vi "Operate.vi"(8 "error in (no error)":errorcluster, 11 "Multiply in":refnum<class "Multiply.lvclass">) -> (0 "error out":errorcluster, 3 "Multiply out":refnum<class "Multiply.lvclass">)   [LabVIEW 2020, in "Multiply.lvclass"]
doc: "This method is used as a child which is used to perform multiplication operation"
uses:
  Multiply.lvclass
  D:/labview/Assignment 24/Math Operations/Math Operations.lvclass
  Multiply.lvclass/Multiply.ctl
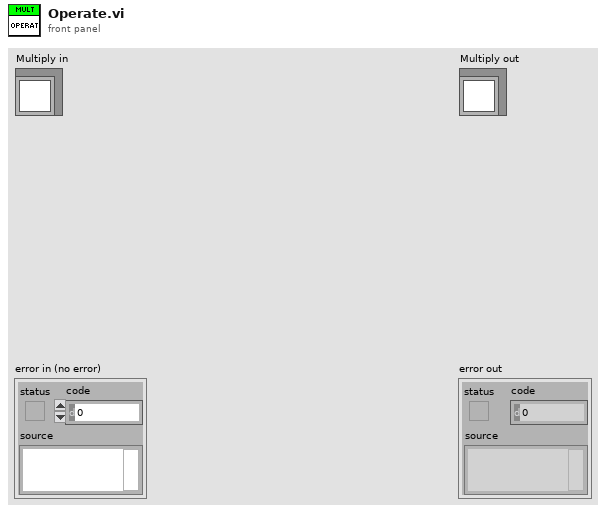
[diagram p1: front panel]
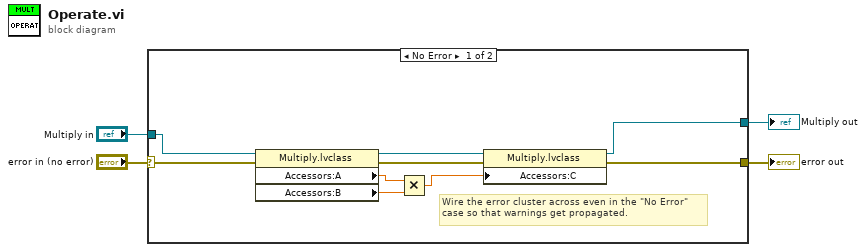
[diagram p0: block diagram]
diagram:
  n1 = case shown="No Error" "error in (no error)" {
    selector: "error in (no error)" -> [w13 w15]
    tunnel: [w6 w15] -> w3
    tunnel: [w5 w14] -> w1
    tunnel: "Multiply in" -> [w11 w14]
    frame No Error {
      # "Wire the error cluster across even in the \"No Error\"\ncase so that warnings get propagated."
      n2 = property class="Multiply.lvclass"(reference=w11, error in=w13) -> (reference out=w10:refnum<class "Multiply.lvclass">, error out=w12:errorcluster, "Accessors:A"=w8:dbl, "Accessors:B"=w9:dbl)
      n3 = Multiply(x=w8, y=w9) -> (x*y=w7:dbl)
      n4 = property class="Multiply.lvclass"(reference=w10, error in=w12, "Accessors:C"=w7) -> (reference out=w5:refnum<class "Multiply.lvclass">, error out=w6:errorcluster)
    }
    frame Error {
    }
  }
  "error out" <- w3
  "Multiply out" <- w1
